vi "Test Update Table for Spartan 5.0.vi"(8 "error in (no error)":errorcluster, 11 "Connection Refnum":T1) -> (0 "error out":errorcluster, 3 "Connection Refnum":T1)   [LabVIEW 2011]
uses:
  Summitek EXT/ODBC/SQL Controls/Connection Refnum.ctl
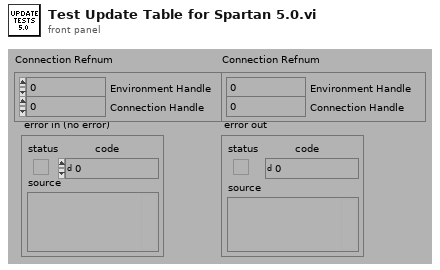
[diagram p1: front panel]
types:
  T1 = typedef "Connection Refnum.ctl" = cluster{"Environment Handle":i32, "Connection Handle":i32}
  T2 = typedef "Statement Refnum.ctl" = cluster{"Statement Handle":i32, "Parameter Number":u16}
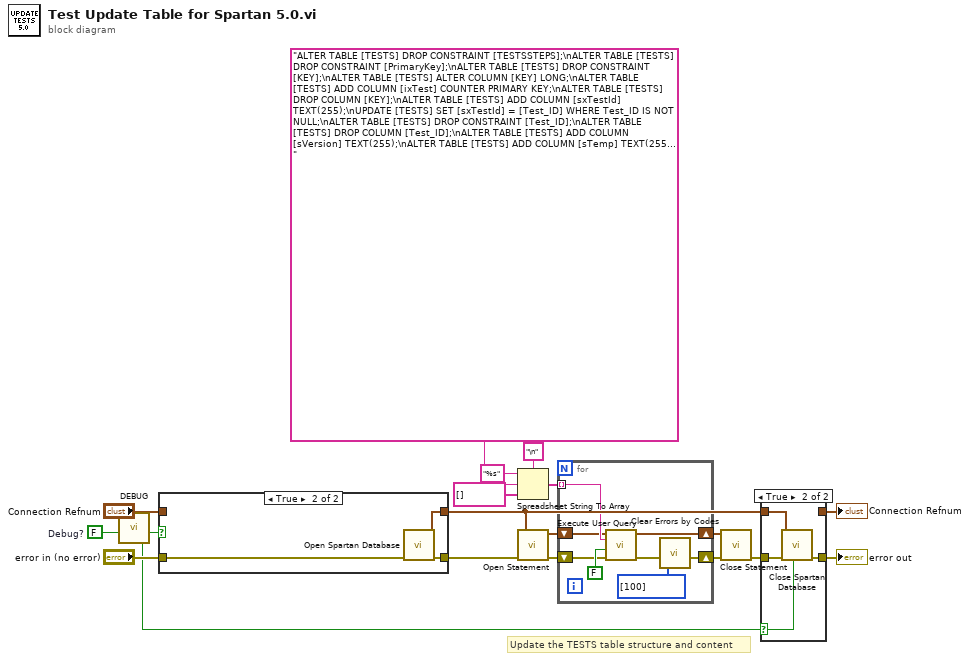
[diagram p0: block diagram]
diagram:
  w10 = FALSE  # Debug?
  # "Update the TESTS table structure and content"
  n1 = call "DEBUG.vi"("Dev DEBUG? (f)"=w10) -> ("DEBUG?"=w9:bool)  [unwired: 1 in, 5 out]
  n2 = case shown="True" w9 {
    tunnel: "Connection Refnum" -> [w20 _]
    tunnel: "error in (no error)" -> [w19 w23]
    tunnel: [w19 w22] -> w11
    tunnel: [w20 w21] -> w7
    frame False {
    }
    frame True {
      n3 = call "Open Spartan Database.vi"("error in (no error)"=w23) -> ("error out"=w22:errorcluster, "Connection Refnum"=w21:T1)  [unwired: 2 in, 7 out]
    }
  }
  n4 = Spreadsheet String To Array(delimiter (Tab)="\n", format string="%s", spreadsheet string="ALTER TABLE [TESTS] DROP CONSTRAINT [TESTSSTEPS];\nALTER TABLE [TESTS] DROP CONSTRAINT [PrimaryKey];\nALTER TABLE [TESTS] DROP CONSTRAINT [KEY];\nALTER TABLE [TESTS] ALTER COLUMN [KEY] LONG;\nALTER TABLE [TESTS] ADD COLUMN [ixTest] COUNTER PRIMARY KEY;\nALTER TABLE [TESTS] DROP COLUMN [KEY];\nALTER TABLE [TESTS] ADD COLUMN [sxTestId] TEXT(255);\nUPDATE [TESTS] SET [sxTestId] = [Test_ID] WHERE Test_ID IS NOT NULL;\nALTER TABLE [TESTS] DROP CONSTRAINT [Test_ID];\nALTER TABLE [TESTS] DROP COLUMN [Test_ID];\nALTER TABLE [TESTS] ADD COLUMN [sVersion] TEXT(255);\nALTER TABLE [TESTS] ADD COLUMN [sTemp] TEXT(255);\nUPDATE [TESTS] SET [sTemp] = [Build];\nALTER TABLE [TESTS] DROP COLUMN [Build];\nUPDATE [TESTS] SET [sVersion] = [Version]+'.'+[sTemp];\nALTER TABLE [TESTS] DROP COLUMN [sTemp];\nALTER TABLE [TESTS] DROP COLUMN [Version];\nALTER TABLE [TESTS] ADD COLUMN [sDriverTypes] TEXT(255);\nUPDATE [TESTS] SET [sDriverTypes] = [DriverTypes];\nALTER TABLE [TESTS] DROP COLUMN [DriverTypes];\nALTER TABLE [TESTS] ADD COLUMN [sDescription] TEXT(255);\nUPDATE [TESTS] SET [sDescription] = [Description];\nALTER TABLE [TESTS] DROP COLUMN [Description];\nALTER TABLE [TESTS] ADD COLUMN [iQuickMode] LONG;\nUPDATE [TESTS] SET [iQuickMode] = [Quickmode];\nALTER TABLE [TESTS] DROP COLUMN [Quickmode];" ("User Query"), array type (2D Dbl)=string[] []) -> (array=w2:string[])
  n5 = call "Open Statement.vi"("error in (no error)"=w11, "Connection Refnum"=w7) -> ("error out"=w6:errorcluster, "Statement Refnum"=w5:T2)  [unwired: 4 out]
  n6 = for {
    shift-right: [w24] -> w3
    shift-left: w6 -> [w28]
    tunnel: w2 -> [w30] mode=indexing
    shift-right: [w27] -> w4
    shift-left: w5 -> [w29]
    n7 = call "Execute User Query.vi"("error in (no error)"=w28, "Return Data? (f)"=FALSE, "User Query"=w30, "Statement Refnum"=w29) -> ("error out"=w25:errorcluster, "Statement Refnum"=w27:T2)  [unwired: 2 out]
    n8 = call "Clear Errors by Codes.vi"("Error Codes\nto Clear (Empty)"=i32[] [100] ("Error Codes\nto Clear (Empty)"), "error in (no error)"=w25) -> ("error out"=w24:errorcluster)  [unwired: 5 out]
  }
  n9 = call "Close Statement.vi"("error in (no error)"=w3, "Statement Refnum"=w4) -> ("error out"=w8:errorcluster)  [unwired: 5 out]
  n10 = case shown="True" w9 {
    selector: w9 -> [_ w34]
    tunnel: w8 -> [w33 w37]
    tunnel: w7 -> [w32 w36]
    tunnel: [w32 _] -> w15
    tunnel: [w33 w35] -> w14
    frame False {
    }
    frame True {
      n11 = call "Close Spartan Database.vi"("Force Close? (f)"=w34, "error in (no error)"=w37, "Connection Refnum"=w36) -> ("error out"=w35:errorcluster)  [unwired: 2 in, 6 out]
    }
  }
  "error out" <- w14
  "Connection Refnum" <- w15
